vi "Monitor VI Position.vi"(11 "VI ref.":refnum<vi>) -> ()   [LabVIEW 2019, in "Window Mover.lvlib"]
doc: "Use the VI to enable panel click-drag behavior on a borderless window. This is an synchronous VI that will continue running as long as the monitored VI is running.\n\nIn most cases, you should not call this VI directly. Instead, use the async. version instead.\n\nYou must provide a VI reference to the VI you wish to monitor."
uses:
  Window Mover.lvlib
  <vilib>/Utility/miscctls.llb/LVRectTypeDef.ctl
  72580d3a-8aca-47bd-b531-ca9c4b92a51b.vi
  <vilib>/Utility/inputDevices.llb/mouseAcquire.vi
  <vilib>/Utility/inputDevices.llb/closeMouse.vi
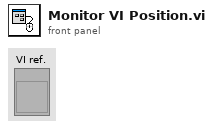
[diagram p1: front panel]
types:
  T1 = typedef "LVRectTypeDef.ctl" = cluster{"Left":i16, "Top":i16, "Right":i16, "Bottom":i16}
  T2 = cluster{"Front Panel.PanelBounds":T1, "axis info":cluster{"Horizontal":i32, "Vertical":i32, "Scrolling":i32}}
  T3 = enum32{"Bad", "Idle", "Run top level", "Running"}
  T4 = cluster{"Horizontal":i32, "Vertical":i32, "Scrolling":i32}
  T5 = cluster{"button 1":bool, "button 2":bool, "button 3":bool, "button 4":bool}
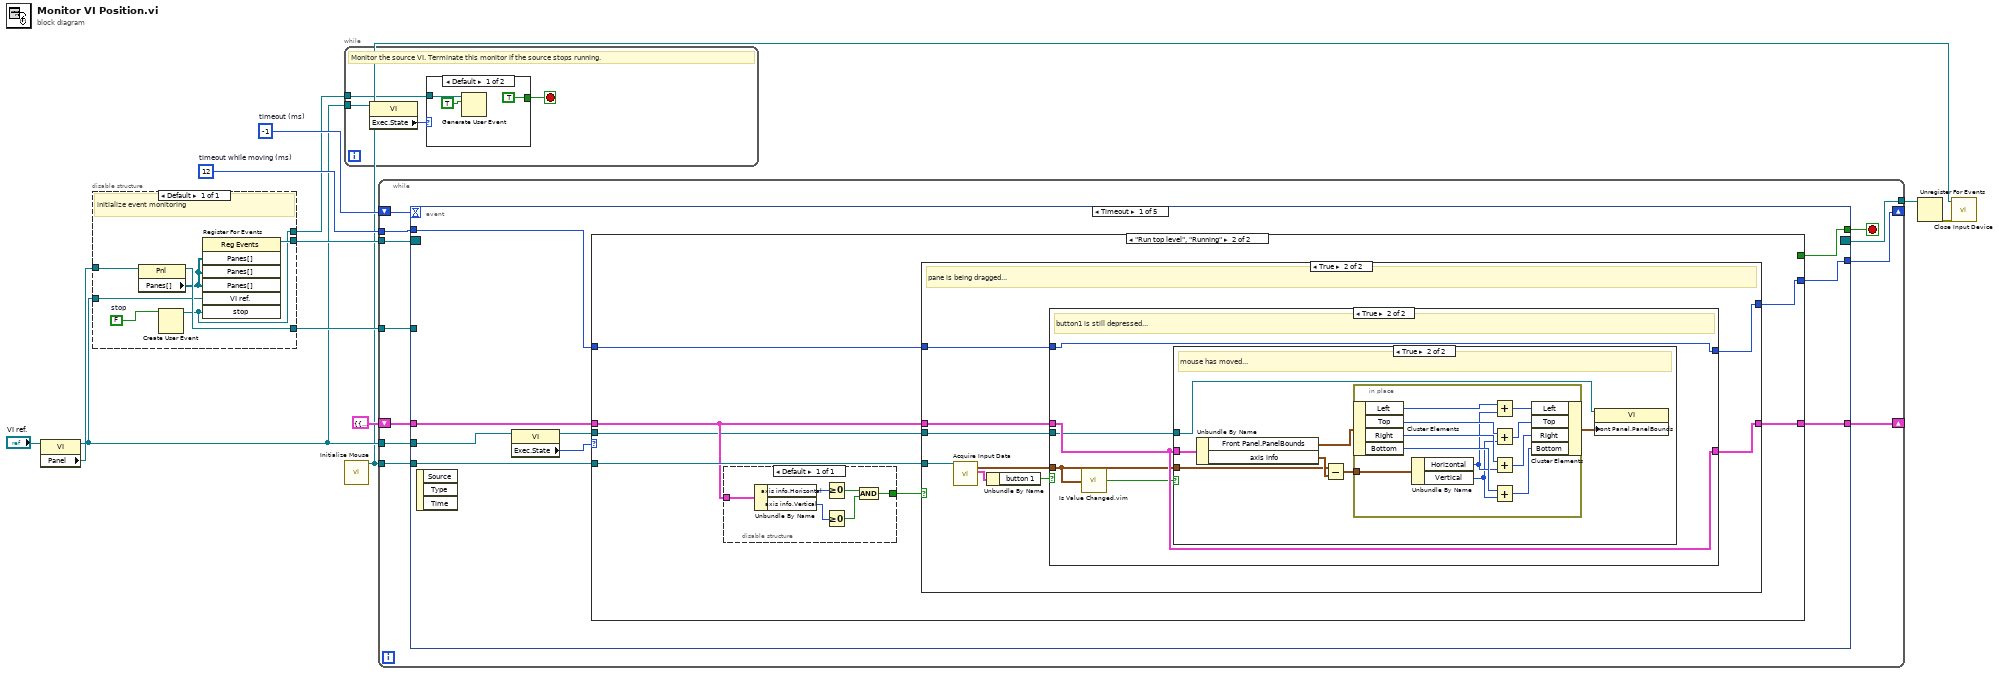
[diagram p0: block diagram]
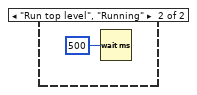
[diagram p2: hidden frame]
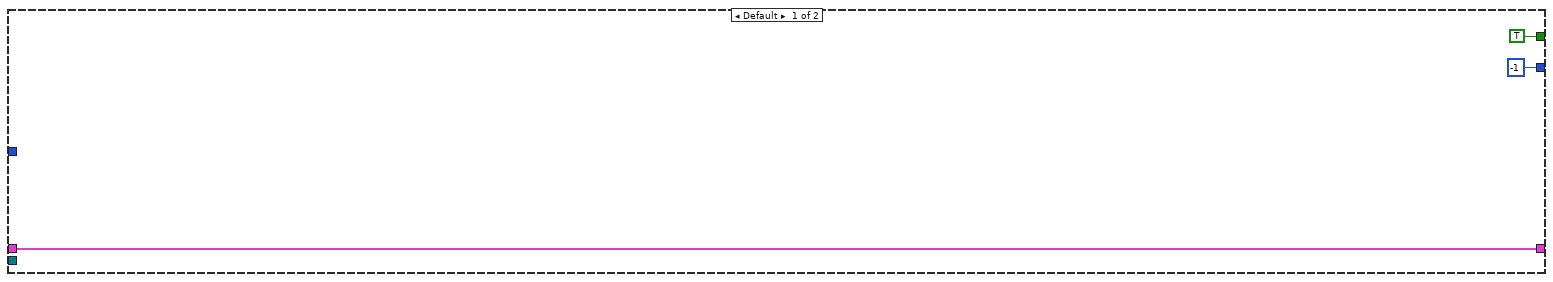
[diagram p3: hidden frame]
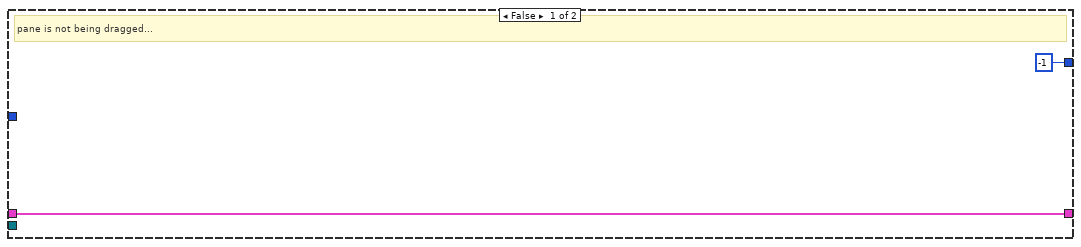
[diagram p4: hidden frame]
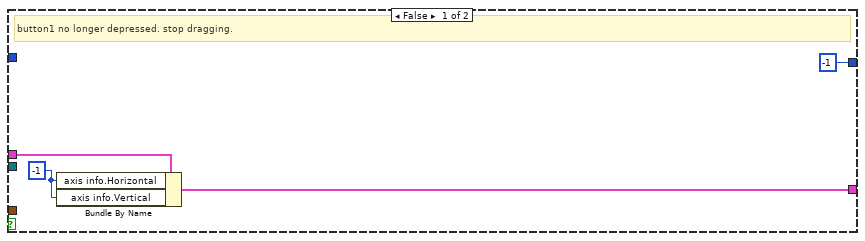
[diagram p5: hidden frame]
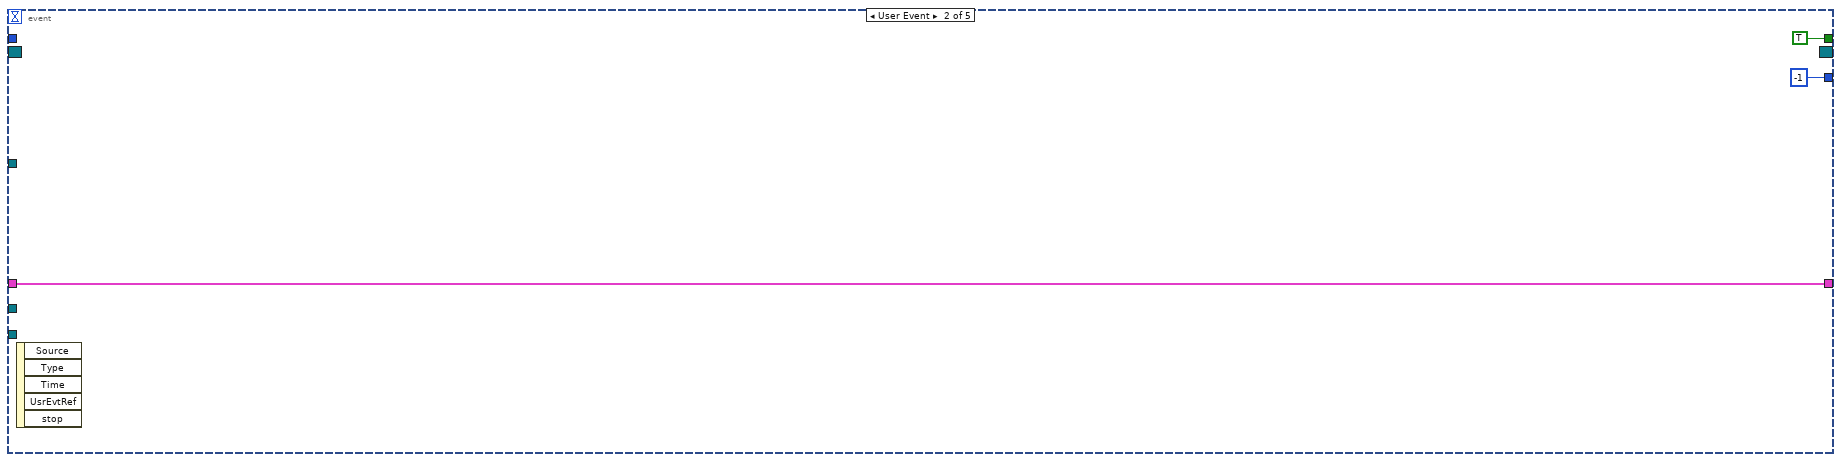
[diagram p7: hidden frame]
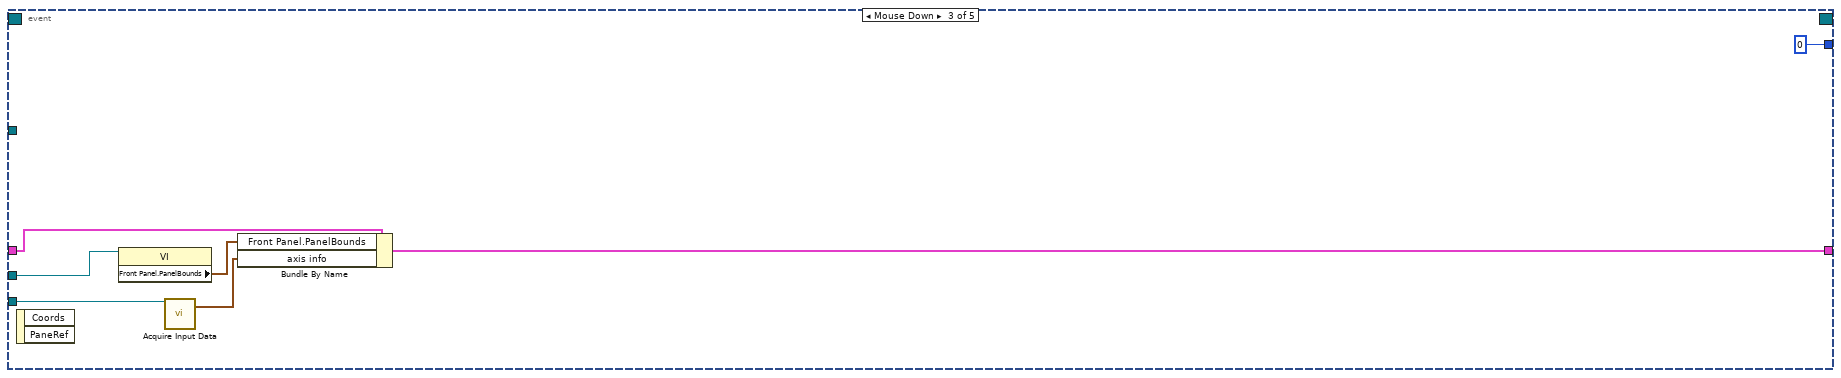
[diagram p8: hidden frame]
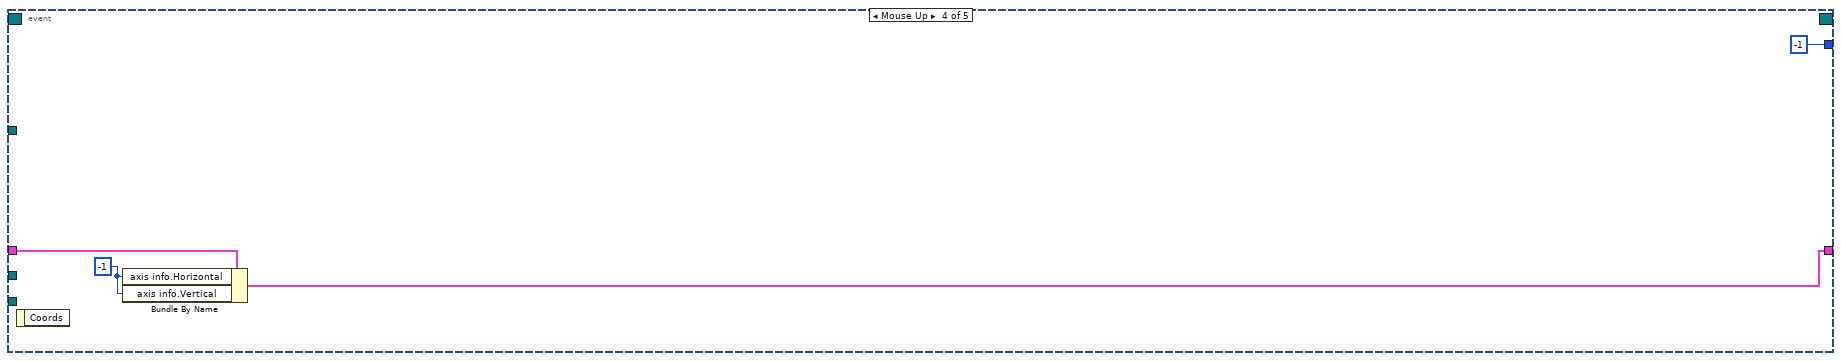
[diagram p9: hidden frame]
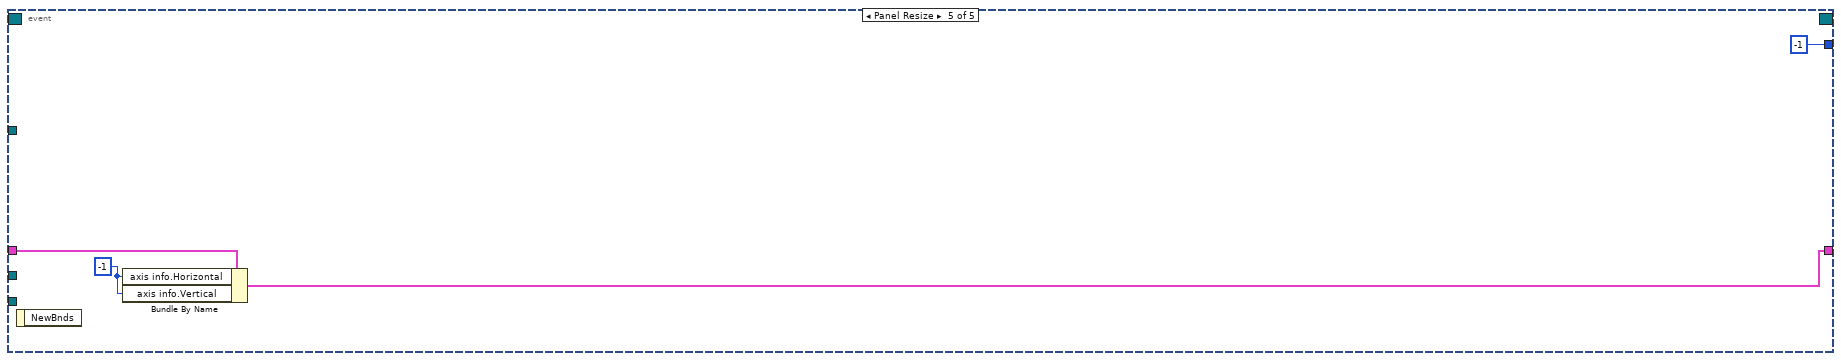
[diagram p10: hidden frame]
diagram:
  w5 = 12  # timeout while moving (ms)
  w6 = -1  # timeout (ms)
  n1 = property class="VI"(reference="VI ref.") -> (reference out=w4:refnum<vi>, "Panel"=w8:refnum<vi>)  [unwired: 1 in, 1 out]
  n2 = disable-structure shown="Default" {
    disable-tunnel: [w19] -> w11
    disable-tunnel: [w18] -> w9
    disable-tunnel: w8 -> [w17]
    disable-tunnel: w4 -> [w15]
    disable-tunnel: [w13] -> w3
    frame Enabled {
      w14 = FALSE  # stop
      # "initialize event monitoring"
      n3 = property class="Pnl"(reference=w17) -> (reference out=w18:refnum<vi>, "Panes[]"=w16:refnum<vi>[])  [unwired: 1 in, 1 out]
      n4 = Create User Event(user event datatype=w14) -> (user event=w13:refnum<user-event>)  [unwired: 1 in, 1 out]
      n5 = register-events(w16, w16, w16, w15, w13) -> (reference out=w19:refnum<event-registration>)  [unwired: 2 in, 1 out]
    }
  }
  n6 = while {
    tunnel: w4 -> [w23]
    tunnel: w3 -> [w20]
    stop <- w21 stop-if-true
    # "Monitor the source VI. Terminate this monitor if the source stops running."
    n7 = property class="VI"(reference=w23) -> ("Exec.State"=w22:T3)  [unwired: 1 in, 2 out]
    n8 = case shown="Default" w22 {
      tunnel: [TRUE _] -> w21
      tunnel: w20 -> [w25 _]
      frame Default {
        n9 = Generate User Event(user event=w25, event data cluster=TRUE ("event data")) -> ()  [unwired: 2 in, 2 out]
      }
      frame "Run top level", "Running" {
        n10 = Wait (ms)(milliseconds to wait=u32 500) -> ()  [unwired: 1 out]
      }
    }
  }
  n11 = call <vilib>:"Initialize Mouse.vi"() -> ("device ID"=w1:refnum<k1>)  [unwired: 10 in, 1 out]
  n12 = while {
    tunnel: w11 -> [w38]
    tunnel: [w37] -> w10
    tunnel: w4 -> [w36]
    tunnel: w1 -> [w34]
    shift-right: [w33] -> _
    shift-left: T2 {"Front Panel.PanelBounds"={"Left"=0, "Top"=0, "Right"=0, "Bottom"=0}, "axis info"={"Horizontal"=0, "Vertical"=0, "Scrolling"=0}} ("output cluster") -> [w32]
    tunnel: w9 -> [w31]
    shift-right: [w29] -> _
    shift-left: w6 -> [w30]
    tunnel: w5 -> [w28]
    stop <- w35 stop-if-true
    n13 = event shown="[0] Timeout" {
      selector: w38 -> [_ _ _ _ _]
      dyn-events: [_ _ _ _ _] -> w37
      timeout: w30 -> [_ _ _ _ _]
      tunnel: w36 -> [w47 _ w106 _ _]
      tunnel: [w45 TRUE _ _ _] -> w35
      tunnel: w34 -> [w44 _ w108 _ _]
      tunnel: [w42 w102 w109 w113 w117] -> w33
      tunnel: w32 -> [w43 w102 w110 w115 w118]
      tunnel: w31 -> [_ _ _ _ _]
      tunnel: [w40 -1 0 -1 -1] -> w29
      tunnel: w28 -> [w39 _ _ _ _]
      event Timeout {
        n14 = event-data() -> ()  [unwired: 1 in, 3 out]
        n15 = property class="VI"(reference=w47) -> (reference out=w41:refnum<vi>, "Exec.State"=w46:T3)  [unwired: 1 in, 1 out]
        n16 = case shown="\"Run top level\", \"Running\"" w46 {
          tunnel: [TRUE _] -> w45
          tunnel: w43 -> [w49 w55]
          tunnel: w44 -> [_ w56]
          tunnel: w41 -> [_ w54]
          tunnel: [w49 w53] -> w42
          tunnel: [-1 w52] -> w40
          tunnel: w39 -> [_ w51]
          frame Default {
          }
          frame "Run top level", "Running" {
            n17 = disable-structure shown="Default" {
              disable-tunnel: w55 -> [w63]
              disable-tunnel: [w58] -> w57
              frame Enabled {
                n18 = Unbundle By Name(w63) -> ("axis info.Horizontal"=w62:i32, "axis info.Vertical"=w61:i32)
                n19 = Greater Or Equal To 0?(x=w62) -> (x >= 0?=w60:bool)
                n20 = Greater Or Equal To 0?(x=w61) -> (x >= 0?=w59:bool)
                n21 = And(x=w60, y=w59) -> (x .and. y?=w58:bool)
              }
            }
            n22 = case shown="True" w57 {
              tunnel: w56 -> [_ w74]
              tunnel: w55 -> [w65 w70]
              tunnel: w54 -> [_ w73]
              tunnel: [w65 w71] -> w53
              tunnel: [-1 w69] -> w52
              tunnel: w51 -> [_ w68]
              frame False {
                # "pane is not being dragged..."
              }
              frame True {
                # "pane is being dragged..."
                n23 = call-poly <vilib>:"Acquire Input Data.vi"("device ID"=w74) -> ("axis info"=w67:T4, "button info"=w72:T5)  [unwired: 15 in, 2 out]
                n24 = Unbundle By Name(w72) -> ("button 1"=w66:bool)
                n25 = case shown="True" w66 {
                  tunnel: w70 -> [w78 w83]
                  tunnel: w67 -> [_ w80]
                  tunnel: w73 -> [_ w82]
                  tunnel: [w77 w83] -> w71
                  tunnel: [-1 ("f") w81] -> w69
                  tunnel: w68 -> [_ w81]
                  frame False {
                    w76 = -1 ("axis info.Horizontal")
                    # "button1 no longer depressed. stop dragging."
                    n26 = Bundle By Name(cluster=w78, "axis info.Horizontal"=w76, "axis info.Vertical"=w76) -> (w77:T2)
                  }
                  frame True {
                    # "button1 is still depressed..."
                    n27 = call "Is Value Changed.vim"("value"=w80) -> ("changed or first call?"=w79:bool)
                    n28 = case shown="True" w79 {
                      tunnel: w83 -> [_ w89]
                      tunnel: w82 -> [_ w85]
                      tunnel: w80 -> [_ w84]
                      frame False {
                        # "mouse has not moved, but button1 is still depressed..."
                      }
                      frame True {
                        # "mouse has moved..."
                        n29 = Unbundle By Name(w89) -> ("Front Panel.PanelBounds"=w88:T1, "axis info"=w90:T4)
                        n30 = Subtract(x=w84, y=w90) -> (x-y=w86:T4)
                        n31 = in-place {
                          in-place-border: w86 -> [w93]
                          n32 = in-place-cluster #1(w88) -> ("Left"=w101:i16, "Top"=w100:i16, "Right"=w99:i16, "Bottom"=w98:i16)
                          n33 = Unbundle By Name(w93) -> ("Horizontal"=w92:i32, "Vertical"=w91:i32)
                          n34 = Add(x=w101, y=w92) -> (x+y=w97:i32)
                          n35 = Add(x=w100, y=w91) -> (x+y=w96:i32)
                          n36 = Add(x=w99, y=w92) -> (x+y=w95:i32)
                          n37 = Add(x=w98, y=w91) -> (x+y=w94:i32)
                          n38 = in-place-cluster #1("Left"=w97, "Top"=w96, "Right"=w95, "Bottom"=w94) -> (w87:T1)
                        }
                        n39 = property class="VI"(reference=w85, "Front Panel.PanelBounds"=w87) -> ()  [unwired: 1 in, 2 out]
                      }
                    }
                  }
                }
              }
            }
          }
        }
      }
      event User Event {
        n40 = event-data() -> ()  [unwired: 1 in, 5 out]
      }
      event Mouse Down {
        n41 = event-data() -> ()  [unwired: 1 in, 2 out]
        n42 = property class="VI"(reference=w106) -> ("Front Panel.PanelBounds"=w105:T1)  [unwired: 1 in, 2 out]
        n43 = call-poly <vilib>:"Acquire Input Data.vi"("device ID"=w108) -> ("axis info"=w107:T4)  [unwired: 15 in, 3 out]
        n44 = Bundle By Name(cluster=w110, "Front Panel.PanelBounds"=w105, "axis info"=w107) -> (w109:T2)
      }
      event Mouse Up {
        w114 = -1 ("axis info.Horizontal")
        n45 = event-data() -> ()  [unwired: 1 in, 1 out]
        n46 = Bundle By Name(cluster=w115, "axis info.Horizontal"=w114, "axis info.Vertical"=w114) -> (w113:T2)
      }
      event Panel Resize {
        w116 = -1 ("axis info.Horizontal")
        n47 = event-data() -> ()  [unwired: 1 in, 1 out]
        n48 = Bundle By Name(cluster=w118, "axis info.Horizontal"=w116, "axis info.Vertical"=w116) -> (w117:T2)
      }
    }
  }
  n49 = Unregister For Events(event registration refnum=w10) -> (error out=w2:errorcluster)  [unwired: 1 in]
  n50 = call-poly <vilib>:"Close Input Device.vi"("error in (no error)"=w2, "device ID"=w1) -> ()  [unwired: 8 in, 1 out]
